vi "Set Enable State on Multiple Controls.vi"(10 "有効?":bool, 11 "制御器":refnum<vi>[](array[refnum])) -> ()   [LabVIEW 2017]
doc: "入力配列のすべての制御器を「有効ステート」値に設定します。"
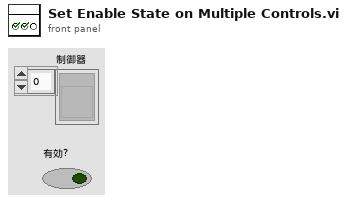
[diagram p1: front panel]
types:
  T1 = enum8{"Enabled", "Disabled", "Disabled and Grayed Out"}
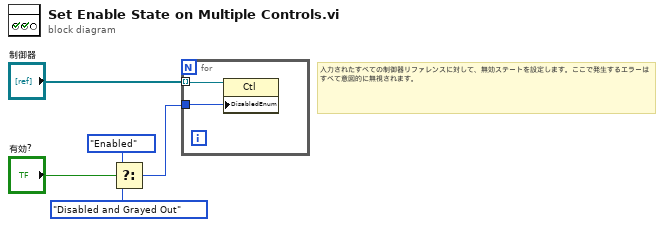
[diagram p0: block diagram]
diagram:
  # "入力されたすべての制御器リファレンスに対して、無効ステートを設定します。ここで発生するエラーはすべて意図的に無視されます。"
  n1 = Select(t=T1."Enabled" ("Disabled"), s="有効?", f=T1."Disabled and Grayed Out" ("Disabled")) -> (s? t:f=w3:T1)
  n2 = for {
    tunnel: "制御器" -> [w7] mode=indexing
    tunnel: w3 -> [w6]
    n3 = property class="Ctl"(reference=w7, "DisabledEnum"=w6) -> ()  [unwired: 1 in, 2 out]
  }
